vi "TiePie_acq_gen.vi"() -> ()   [LabVIEW 2021]
uses:
  hs3.dll
panel:
  out "Transmitted  Waveform":u16[](graph)
  out "Recieved Samples":i32
  out "Array":string[](array[string])
  out "Recieved Message":string
  in  "Expected Characters":u16
  out "Actual Message Duration":dbl=0.4
  in  "Tranmission Message":string="A"
  in  "Inputs":T1={"Frequency1"=2000.0, "Bit Duration in ms"=0.05, "Frequency2"=4000.0, "Amplitude Scale"=1.0, "Sampling Rate"=50000} {"Frequency2" format="%#_13g"; "Frequency1" format="%#_13g"}
  out "Total Message Duration":dbl=0.4
  in  "Amplitude":dbl(slide)=0.99 min=0.01 max=12.0 step=0.01 scale=0.01..12.0
  in  "Gen_SignalType":u16(ring)=5 caption="Type Signal" items=["Sinus", "Triangle", "Carré", "DC", "Bruit", "Arbitrary"]
  in  "Offset":dbl(slide)=6.661338147750939e-16 min=-12.0 max=12.0 step=0.1 scale=-6.0..6.0
  in  "Démarrer Générateur":bool
  out "Memo untrig":bool
  out "Untrigged":bool
  out "Timebase [s]":dbl=1e-07
  in  "Level [V]":dbl min=-80.0 max=80.0 step=0.001
  in  "Direction":u16(ring) items=["Rising", "Falling"]
  in  "CH1 : AC/DC":u16(ring)=1 items=["AC", "DC"]
  in  "CH2 : AC/DC":u16(ring)=1 items=["AC", "DC"]
  in  "No. of samples":u32=20000 min=100 max=130000 step=1
  in  "Source":u16(ring)=14 items=["CH1"=0, "CH2"=1, "None"=9, "Gen"=14]
  in  "Hysteresis [V]":sgl=0.039997473 min=-100 max=100 step=0.0001 format="%#.4f"
  in  "Active Channel":u16(ring)=1 items=["CH1"=1, "CH2"=2, "CH1 + CH2"=3]
  in  "CH1 Range":dbl(ring)=2.0 items=["200mV"=0.2, "400mV"=0.4, "800mV"=0.8, "2V"=2.0, "4V"=4.0, "8V"=8.0, "20V"=20.0, "40V"=40.0, "80V"=80.0]
  in  "CH2 Range":dbl(ring)=8.0 items=["200mV"=0.2, "400mV"=0.4, "800mV"=0.8, "2V"=2.0, "4V"=4.0, "8V"=8.0, "20V"=20.0, "40V"=40.0, "80V"=80.0]
  in  "Postsamples":i32 min=0 max=130000 step=1
  out "DataReady":bool
  out "Measuring":bool
  in  "Démarrer Acquisition/\nStart Acquisition":bool
  out "Channel B":dbl[](graph)
  out "Channel A":dbl[](graph)
  out "init A":dbl[](array[numeric])
  out "init B":dbl[](array[numeric])
  out "S/N":u32
  out "TiePie OK":bool
  # "General"
  # "Trigger settings"
  # "Canal 1"
  # "Canal 2"
  # "For Debugging"
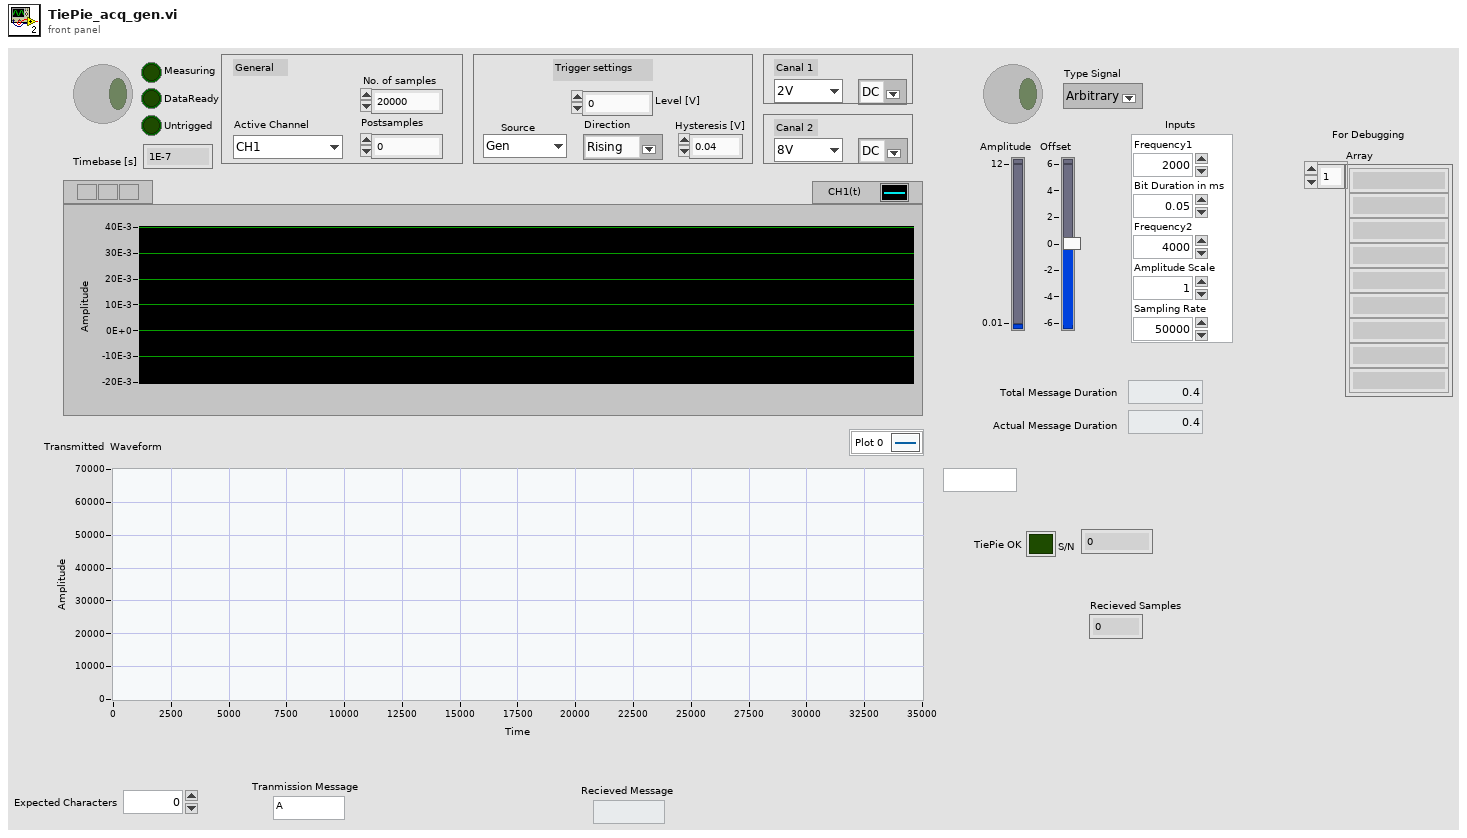
[diagram p1: front panel]
types:
  T1 = cluster{"Frequency1":dbl, "Bit Duration in ms":dbl, "Frequency2":dbl, "Amplitude Scale":dbl, "Sampling Rate":u32}
  T2 = enum8{"Enabled", "Disabled", "Disabled and Grayed Out"}
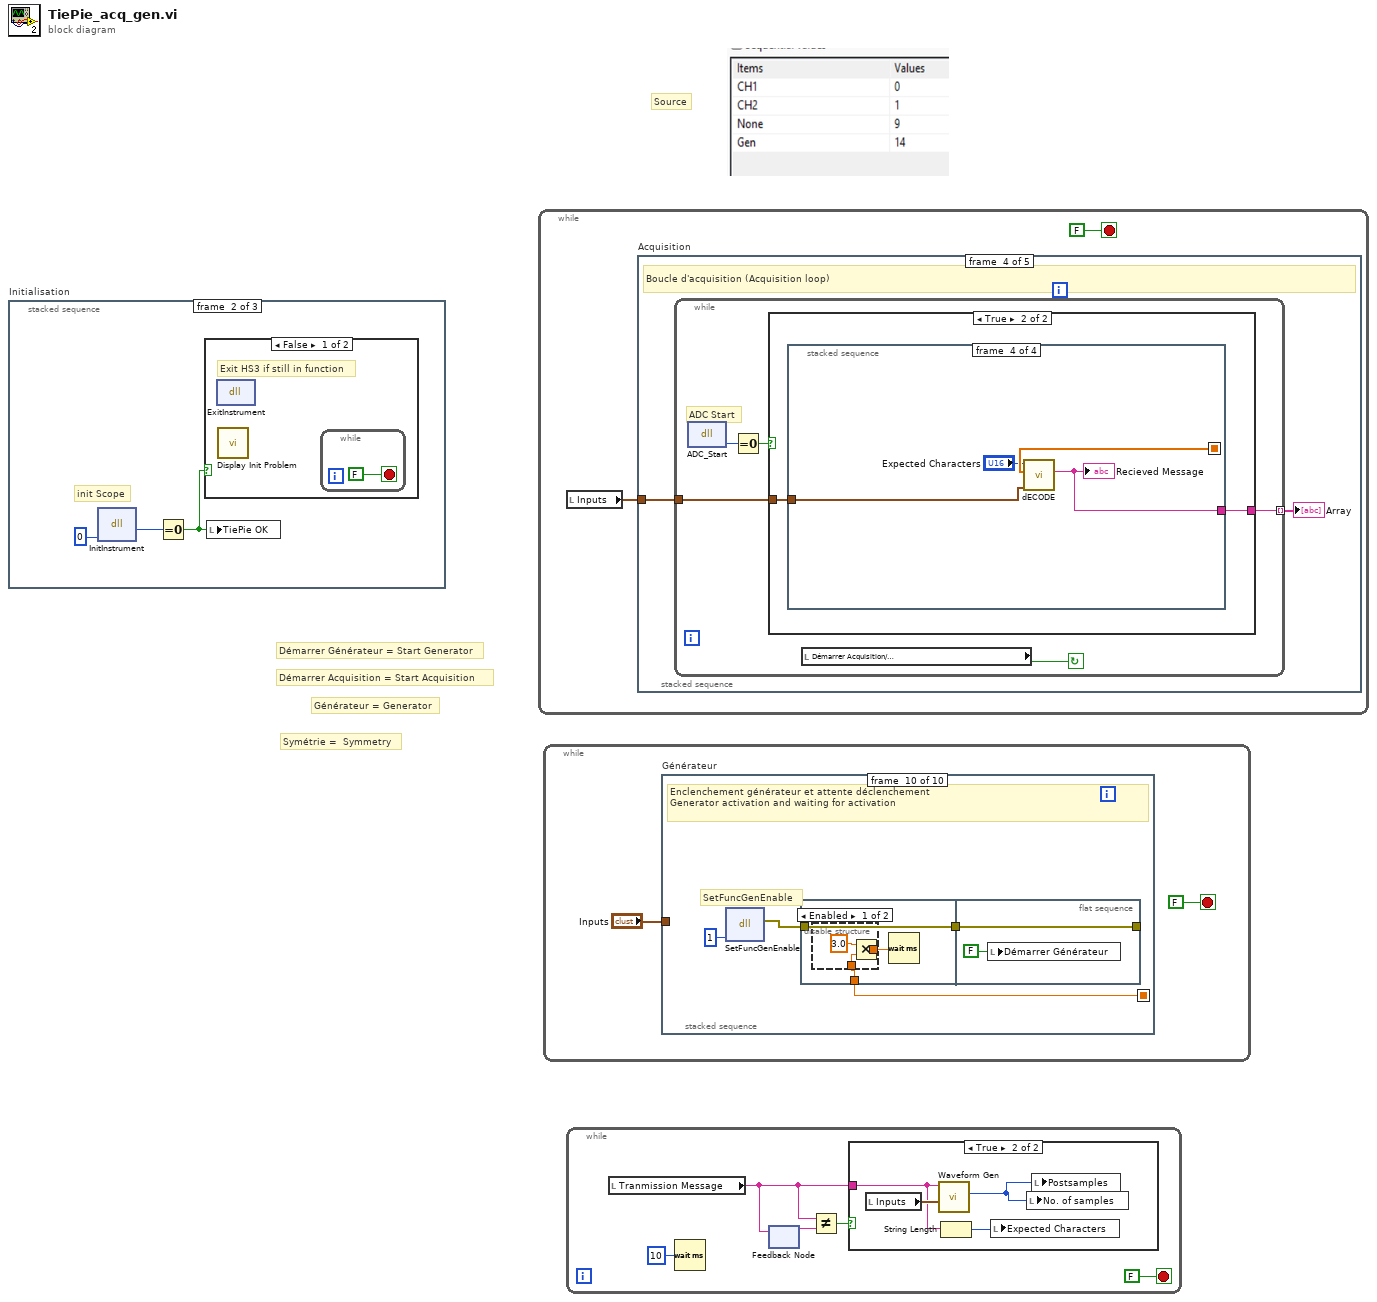
[diagram p0: block diagram]
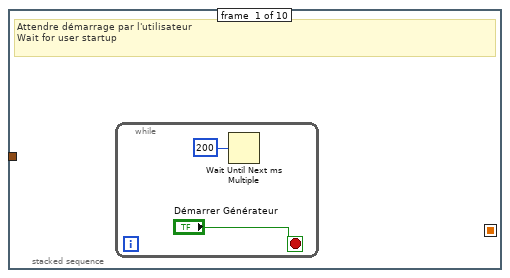
[diagram p3: hidden frame]
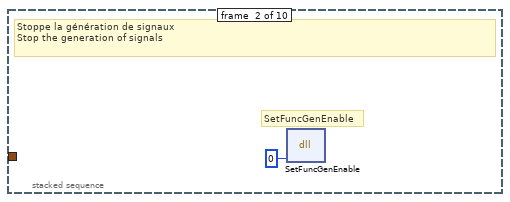
[diagram p4: hidden frame]
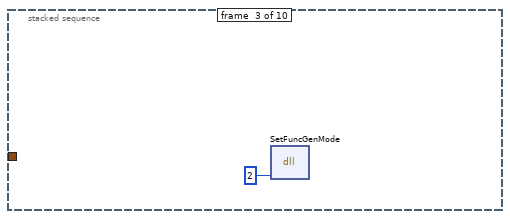
[diagram p5: hidden frame]
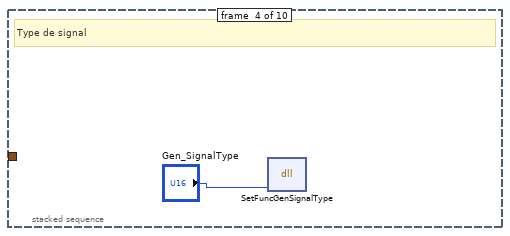
[diagram p6: hidden frame]
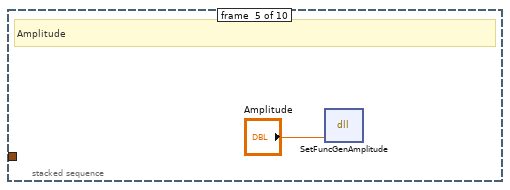
[diagram p7: hidden frame]
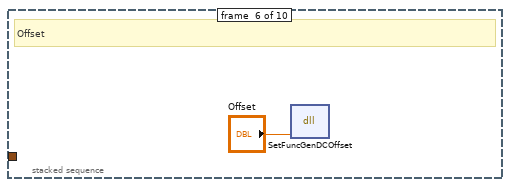
[diagram p8: hidden frame]
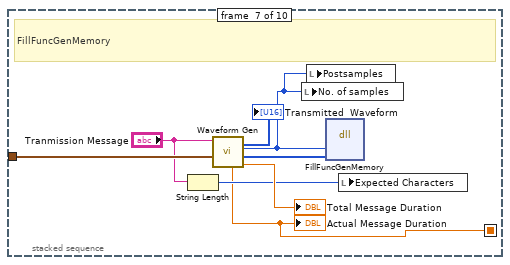
[diagram p9: hidden frame]
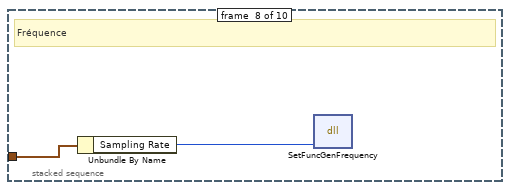
[diagram p10: hidden frame]
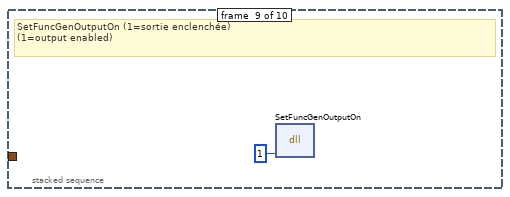
[diagram p11: hidden frame]
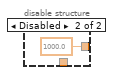
[diagram p12: hidden frame]
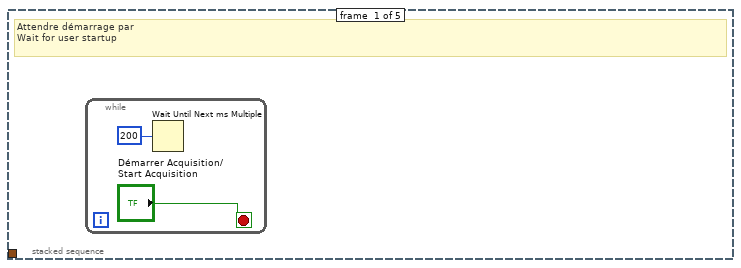
[diagram p13: hidden frame]
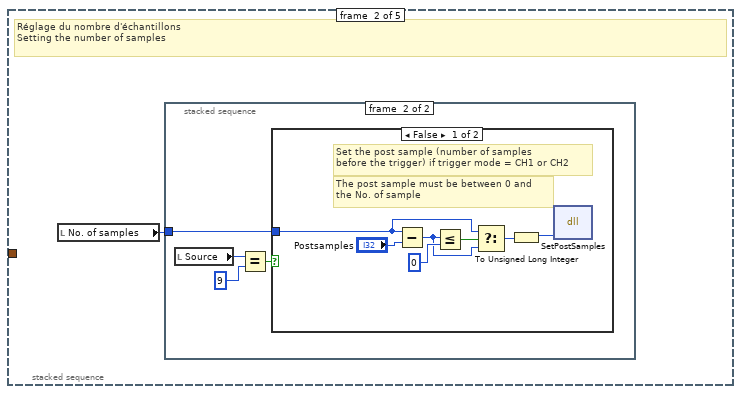
[diagram p14: hidden frame]
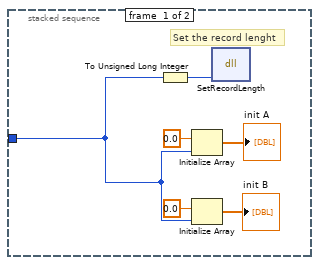
[diagram p15: hidden frame]
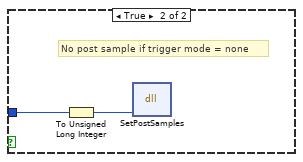
[diagram p16: hidden frame]
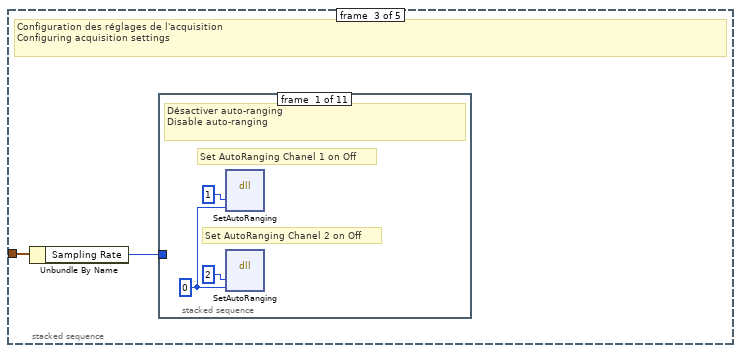
[diagram p17: hidden frame]
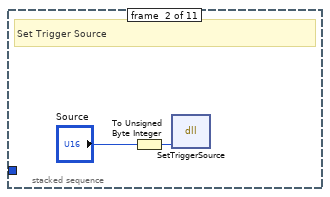
[diagram p18: hidden frame]
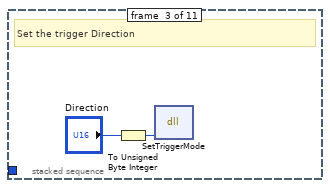
[diagram p19: hidden frame]
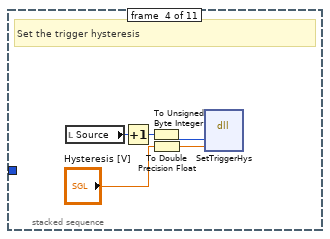
[diagram p20: hidden frame]
diagram:
  # "Source"
  # "Symétrie =  Symmetry"
  # "Générateur = Generator"
  # "Démarrer Acquisition = Start Acquisition"
  # "Démarrer Générateur = Start Generator"
  n1 = stacked-sequence "Initialisation" {
    frame #0 {
      n2 = local write "Démarrer Acquisition/\nStart Acquisition"(FALSE ("Démarrer Acquisition")) -> ()
      n3 = local write "Démarrer Générateur"(FALSE ("Démarrer")) -> ()
      n4 = Wait (ms)(milliseconds to wait=u32 200 ("attente (ms)")) -> ()  [unwired: 1 out]
      n5 = property on="Démarrer Acquisition/\nStart Acquisition" class="Bool (strict)"("DisabledEnum"=T2."Disabled and Grayed Out" ("Désactivé")) -> ()  [unwired: 2 in, 2 out]
      n6 = property on="Démarrer Générateur" class="Bool (strict)"("DisabledEnum"=T2."Disabled and Grayed Out" ("Désactivé")) -> ()  [unwired: 2 in, 2 out]
      "TiePie OK" <- FALSE ("Scope\n init")
      "S/N" <- u32 0 ("Serialnumber")
      "DataReady" <- FALSE ("DataReady")
      "Measuring" <- FALSE ("Measuring")
      "Untrigged" <- FALSE ("Untrigged")
    }
    frame #1 {
      # "init Scope"
      n7 = dll-call lib="C:/Users/BD2QHB4/Desktop/Hassanullah khan/hs3.dll" fn="InitInstrument"("wAddress"=u16 0) -> (w12:u16)  [unwired: 4 in, 2 out]
      n8 = Equal To 0?(x=w12) -> (x = 0?=w11:bool)
      n9 = case shown="False" w11 {
        frame False {
          # "Exit HS3 if still in function"
          n10 = dll-call lib="C:/Users/BD2QHB4/Desktop/Hassanullah khan/hs3.dll" fn="ExitInstrument"() -> ()  [unwired: 4 in, 2 out]
          n11 = call "Display Init Problem"() -> ()  [unwired: 10 in, 2 out]
          n12 = while {
            stop <- FALSE stop-if-true
          }
        }
        frame True {
        }
      }
      n13 = local write "TiePie OK"(w11) -> ()
    }
    frame #2 {
      n14 = local read "S/N"() -> (w17:u32)
      n15 = property on="Démarrer Acquisition/\nStart Acquisition" class="Bool (strict)"("DisabledEnum"=T2."Enabled" ("Désactivé")) -> ()  [unwired: 2 in, 2 out]
      n16 = property on="Démarrer Générateur" class="Bool (strict)"("DisabledEnum"=T2."Enabled" ("Désactivé")) -> ()  [unwired: 2 in, 2 out]
      n17 = dll-call lib="C:/Users/BD2QHB4/Desktop/Hassanullah khan/hs3.dll" fn="GetSerialNumber"("dwSerialNumber"=w17) -> ("dwSerialNumber"=w18:u32)  [unwired: 4 in, 2 out]
      n18 = local write "S/N"(w18) -> ()
    }
  }
  n19 = while {
    stop <- FALSE stop-if-true
    n20 = local read "Inputs"() -> (w19:T1)
    n21 = stacked-sequence "Acquisition" {
      tunnel: w19 -> [_ _ w44 w81 _]
      frame #0 {
        # "Attendre démarrage par \nWait for user startup"
        n22 = while {
          stop <- "Démarrer Acquisition/\nStart Acquisition" stop-if-true
          n23 = Wait Until Next ms Multiple(millisecond multiple=u32 200) -> ()  [unwired: 1 out]
        }
      }
      frame #1 {
        # "Réglage du nombre d'échantillons\nSetting the number of samples"
        n24 = local read "No. of samples"() -> (w23:u32)
        n25 = stacked-sequence {
          tunnel: w23 -> [w24 w30]
          frame #0 {
            # "Set the record lenght"
            n26 = To Unsigned Long Integer(number=w24) -> (unsigned 32bit integer=w29:u32)
            n27 = Initialize Array(0.0, w24) -> (→"init A":dbl[])
            n28 = Initialize Array(0.0, w24) -> (→"init B":dbl[])
            n29 = dll-call lib="C:/Users/BD2QHB4/Desktop/Hassanullah khan/hs3.dll" fn="SetRecordLength"("dTotal"=w29) -> ()  [unwired: 5 in, 2 out]
          }
          frame #1 {
            n30 = local read "Source"() -> (w33:u16)
            n31 = Equal?(x=w33, y=u16 9) -> (x = y?=w31:bool)
            n32 = case shown="False" w31 {
              tunnel: w30 -> [w36 w42]
              frame False {
                # "The post sample must be between 0 and \nthe No. of sample"
                # "Set the post sample (number of samples\nbefore the trigger) if trigger mode = CH1 or CH2"
                n33 = Subtract(x=w36, y="Postsamples") -> (x-y=w35:u32)
                n34 = Less Or Equal?(x=w35, y=0) -> (x <= y?=w37:bool)
                n35 = Select(t=w36, s=w37, f=w35) -> (s? t:f=w39:u32)
                n36 = To Unsigned Long Integer(number=w39) -> (unsigned 32bit integer=w40:u32)
                n37 = dll-call lib="C:/Users/BD2QHB4/Desktop/Hassanullah khan/hs3.dll" fn="SetPostSamples"("dTotal"=w40) -> ()  [unwired: 5 in, 2 out]
              }
              frame True {
                # "No post sample if trigger mode = none"
                n38 = To Unsigned Long Integer(number=w42) -> (unsigned 32bit integer=w41:u32)
                n39 = dll-call lib="C:/Users/BD2QHB4/Desktop/Hassanullah khan/hs3.dll" fn="SetPostSamples"("dTotal"=w41) -> ()  [unwired: 5 in, 2 out]
              }
            }
          }
        }
      }
      frame #2 {
        # "Configuration des réglages de l'acquisition\nConfiguring acquisition settings"
        n40 = Unbundle By Name(w44) -> ("Sampling Rate"=w43:u32)
        n41 = stacked-sequence {
          tunnel: w43 -> [_ _ _ _ _ _ _ _ _ _ w76]
          frame #0 {
            w47 = u8 0
            # "Set AutoRanging Chanel 1 on Off"
            # "Set AutoRanging Chanel 2 on Off"
            # "Désactiver auto-ranging\nDisable auto-ranging"
            n42 = dll-call lib="C:/Users/BD2QHB4/Desktop/Hassanullah khan/hs3.dll" fn="SetAutoRanging"("byCh"=u8 1, "byMode"=w47) -> ()  [unwired: 6 in, 2 out]
            n43 = dll-call lib="C:/Users/BD2QHB4/Desktop/Hassanullah khan/hs3.dll" fn="SetAutoRanging"("byCh"=u8 2, "byMode"=w47) -> ()  [unwired: 6 in, 2 out]
          }
          frame #1 {
            # "Set Trigger Source"
            n44 = To Unsigned Byte Integer(number="Source") -> (unsigned 8bit integer=w49:u8)
            n45 = dll-call lib="C:/Users/BD2QHB4/Desktop/Hassanullah khan/hs3.dll" fn="SetTriggerSource"("byTrigSource"=w49) -> ()  [unwired: 5 in, 2 out]
          }
          frame #2 {
            # "Set the trigger Direction"
            n46 = To Unsigned Byte Integer(number="Direction") -> (unsigned 8bit integer=w51:u8)
            n47 = dll-call lib="C:/Users/BD2QHB4/Desktop/Hassanullah khan/hs3.dll" fn="SetTriggerMode"("byTrigMode"=w51) -> ()  [unwired: 5 in, 2 out]
          }
          frame #3 {
            # "Set the trigger hysteresis"
            n48 = local read "Source"() -> (w55:u16)
            n49 = Increment(x=w55) -> (x+1=w53:u16)
            n50 = To Unsigned Byte Integer(number=w53) -> (unsigned 8bit integer=w56:u8)
            n51 = To Double Precision Float(number="Hysteresis [V]") -> (double precision float=w54:dbl)
            n52 = dll-call lib="C:/Users/BD2QHB4/Desktop/Hassanullah khan/hs3.dll" fn="SetTriggerHys"("byCh"=w56, "rHysteresis"=w54) -> ()  [unwired: 6 in, 2 out]
          }
          frame #4 {
            # "Set the trigger Level"
            n53 = local read "Source"() -> (w60:u16)
            n54 = Increment(x=w60) -> (x+1=w58:u16)
            n55 = To Unsigned Byte Integer(number=w58) -> (unsigned 8bit integer=w61:u8)
            n56 = To Double Precision Float(number="Level [V]") -> (double precision float=w59:dbl)
            n57 = dll-call lib="C:/Users/BD2QHB4/Desktop/Hassanullah khan/hs3.dll" fn="SetTriggerLevel"("byCh"=w61, "rLvl"=w59) -> ()  [unwired: 6 in, 2 out]
          }
          frame #5 {
            # "Set the mesure mode (Source)"
            n58 = To Unsigned Byte Integer(number="Active Channel") -> (unsigned 8bit integer=w63:u8)
            n59 = dll-call lib="C:/Users/BD2QHB4/Desktop/Hassanullah khan/hs3.dll" fn="SetMeasureMode"("byMode"=w63) -> ()  [unwired: 5 in, 2 out]
          }
          frame #6 {
            # "Set the channel 1 Range"
            n60 = To Double Precision Float(number="CH1 Range") -> (double precision float=w66:dbl)
            n61 = dll-call lib="C:/Users/BD2QHB4/Desktop/Hassanullah khan/hs3.dll" fn="SetSensitivity"("byCh"=u8 1, "rSens"=w66) -> ()  [unwired: 6 in, 2 out]
          }
          frame #7 {
            # "Set the channel 2 Range"
            n62 = To Double Precision Float(number="CH2 Range") -> (double precision float=w68:dbl)
            n63 = dll-call lib="C:/Users/BD2QHB4/Desktop/Hassanullah khan/hs3.dll" fn="SetSensitivity"("byCh"=u8 2, "rSens"=w68) -> ()  [unwired: 6 in, 2 out]
          }
          frame #8 {
            # "Set the coupling CH1"
            n64 = To Unsigned Byte Integer(number="CH1 : AC/DC") -> (unsigned 8bit integer=w71:u8)
            n65 = dll-call lib="C:/Users/BD2QHB4/Desktop/Hassanullah khan/hs3.dll" fn="SetCoupling"("byCh"=u8 1, "byMode"=w71) -> ()  [unwired: 6 in, 2 out]
          }
          frame #9 {
            # "Set the coupling CH2"
            n66 = To Unsigned Byte Integer(number="CH2 : AC/DC") -> (unsigned 8bit integer=w75:u8)
            n67 = dll-call lib="C:/Users/BD2QHB4/Desktop/Hassanullah khan/hs3.dll" fn="SetCoupling"("byCh"=u8 2, "byMode"=w75) -> ()  [unwired: 6 in, 2 out]
          }
          frame #10 {
            # "Set the sample frequency"
            n68 = To Unsigned Long Integer(number=w76) -> (unsigned 32bit integer=w79:u32)
            n69 = dll-call lib="C:/Users/BD2QHB4/Desktop/Hassanullah khan/hs3.dll" fn="SetSampleFrequency"("dFreq"=w79) -> ("dFreq"=w78:u32)  [unwired: 4 in, 2 out]
            n70 = Reciprocal(x=w78) -> (1/x=w77:dbl)
            "Timebase [s]" <- w77
            n71 = property on="Channel A" class="WFGraph (strict)"("XScale.Multiplier"=w77) -> ()  [unwired: 2 in, 2 out]
            n72 = property on="Channel B" class="WFGraph (strict)"("XScale.Multiplier"=w77) -> ()  [unwired: 2 in, 2 out]
          }
        }
      }
      frame #3 {
        # "Boucle d'acquisition (Acquisition loop)"
        n73 = while {
          tunnel: w81 -> [w83]
          tunnel: [w82] -> w80 mode=indexing
          stop <- w84 continue-if-true
          # "ADC Start"
          n74 = dll-call lib="C:/Users/BD2QHB4/Desktop/Hassanullah khan/hs3.dll" fn="ADC_Start"() -> (w86:u16)  [unwired: 3 in, 2 out]
          n75 = Equal To 0?(x=w86) -> (x = 0?=w85:bool)
          n76 = case shown="True" w85 {
            tunnel: w83 -> [_ w89]
            tunnel: [_ w88] -> w82
            frame False {
              # "ACQ problem display"
              n77 = call "Affiche problème ACQ"() -> ()  [unwired: 10 in, 2 out]
              n78 = while {
                stop <- FALSE stop-if-true
              }
            }
            frame True {
              n79 = stacked-sequence {
                seq-local: [_ _ w104 _] -> [_ _ _ w112]
                tunnel: w89 -> [_ _ _ w110]
                tunnel: [_ _ _ w109] -> w88
                frame #0 {
                  # "ADC_Running"
                  # "Mesure en cours\nAction in progress"
                  n80 = dll-call lib="C:/Users/BD2QHB4/Desktop/Hassanullah khan/hs3.dll" fn="ADC_Running"() -> ("type de retour"=w93:u16)  [unwired: 3 in, 2 out]
                  n81 = Equal?(x=u16 1, y=w93) -> (x = y?=w92:bool)
                  n82 = local write "Measuring"(w92) -> ()
                  "Memo untrig" <- FALSE ("Memo untrig")
                }
                frame #1 {
                  # "Attendre mesure prête (ou timeout trigger)\nWait for measurement ready (or timeout trigger)"
                  n83 = while {
                    i -> [w98]
                    stop <- w95 stop-if-true
                    n84 = Equal To 0?(x=w98) -> (x = 0?=w97:bool)
                    n85 = call "Temps écoulé"("Time Target (s)"=1.0, "Reset"=w97, "Auto Reset"=FALSE) -> ("Time has Elapsed"=w94:bool)  [unwired: 9 in, 7 out]
                    n86 = case shown="True" w94 {
                      selector: w94 -> [w102 _]
                      frame True {
                        # "Force Trig"
                        n87 = dll-call lib="C:/Users/BD2QHB4/Desktop/Hassanullah khan/hs3.dll" fn="ADC_ForceTrig"() -> ()  [unwired: 4 in, 2 out]
                        n88 = local write "Memo untrig"(w102) -> ()
                      }
                      frame False {
                      }
                    }
                    n89 = dll-call lib="C:/Users/BD2QHB4/Desktop/Hassanullah khan/hs3.dll" fn="ADC_Ready"() -> (w96:u16)  [unwired: 3 in, 2 out]
                    n90 = Greater Than 0?(x=w96) -> (x > 0?=w95:bool)
                    n91 = local write "DataReady"(w95) -> ()
                    n92 = Wait Until Next ms Multiple(millisecond multiple=u32 5) -> ()  [unwired: 1 out]
                  }
                }
                frame #2 {
                  # "Get ADC Value in Volt"
                  # "Récupération des valeurs\nRetrieving values"
                  n93 = local read "Memo untrig"() -> (w105:bool)
                  n94 = local read "init A"() -> (w107:dbl[])
                  n95 = local read "init B"() -> (w108:dbl[])
                  n96 = local write "Untrigged"(w105) -> ()
                  n97 = dll-call lib="C:/Users/BD2QHB4/Desktop/Hassanullah khan/hs3.dll" fn="ADC_GetDataVolt"("dCh1"=w107, "dCh2"=w108) -> ("dCh1"=w104:dbl[], "dCh2"=→"Channel B":dbl[])  [unwired: 4 in, 2 out]
                  "Channel A" <- w104
                  n98 = Array Size(array=w104) -> (size(s)=→"Recieved Samples":i32)
                }
                frame #3 {
                  n99 = call "dECODE.vi"("Inputs"=w110, "Waveform Array"=w112, "Expected Characters"="Expected Characters") -> ("string"=w109:string)  [unwired: 8 in]
                  "Recieved Message" <- w109
                }
              }
            }
          }
          n100 = local read "Démarrer Acquisition/\nStart Acquisition"() -> (w84:bool)
        }
        "Array" <- w80
      }
      frame #4 {
        # "ADC_Running"
        # "ADC_abort"
        # "Stoppe l'acquisition\nStop the acquisition"
        n101 = dll-call lib="C:/Users/BD2QHB4/Desktop/Hassanullah khan/hs3.dll" fn="ADC_Running"() -> ("type de retour"=w114:u16)  [unwired: 3 in, 2 out]
        n102 = dll-call lib="C:/Users/BD2QHB4/Desktop/Hassanullah khan/hs3.dll" fn="ADC_Abort"() -> ()  [unwired: 4 in, 2 out]
        n103 = Equal?(x=u16 1, y=w114) -> (x = y?=w115:bool)
        n104 = local write "DataReady"(FALSE ("DataReady")) -> ()
        n105 = local write "Measuring"(w115) -> ()
      }
    }
  }
  n106 = while {
    stop <- FALSE stop-if-true
    n107 = stacked-sequence "Générateur" {
      seq-local: [_ _ _ _ _ _ w126 _ _ _] -> [_ _ _ _ _ _ _ _ _ w137]
      tunnel: "Inputs" -> [_ _ _ _ _ _ w132 w135 _ _]
      frame #0 {
        # "Attendre démarrage par l'utilisateur\nWait for user startup"
        n108 = while {
          stop <- "Démarrer Générateur" stop-if-true
          n109 = Wait Until Next ms Multiple(millisecond multiple=u32 200) -> ()  [unwired: 1 out]
        }
      }
      frame #1 {
        # "SetFuncGenEnable"
        # "Stoppe la génération de signaux\nStop the generation of signals"
        n110 = dll-call lib="C:/Users/BD2QHB4/Desktop/Hassanullah khan/hs3.dll" fn="SetFuncGenEnable"("arg1"=u16 0) -> ()  [unwired: 5 in, 2 out]
      }
      frame #2 {
        n111 = dll-call lib="C:/Users/BD2QHB4/Desktop/Hassanullah khan/hs3.dll" fn="SetFuncGenMode"("dwMode"=2) -> ()  [unwired: 5 in, 2 out]
      }
      frame #3 {
        # "Type de signal"
        n112 = dll-call lib="C:/Users/BD2QHB4/Desktop/Hassanullah khan/HS3.dll" fn="SetFuncGenSignalType"("SignalType"="Gen_SignalType") -> ()  [unwired: 5 in, 2 out]
      }
      frame #4 {
        # "Amplitude"
        n113 = dll-call lib="C:/Users/BD2QHB4/Desktop/Hassanullah khan/hs3.dll" fn="SetFuncGenAmplitude"("Amplitude") -> ()  [unwired: 5 in, 2 out]
      }
      frame #5 {
        # "Offset"
        n114 = dll-call lib="C:/Users/BD2QHB4/Desktop/Hassanullah khan/HS3.dll" fn="SetFuncGenDCOffset"("Offset") -> ()  [unwired: 5 in, 2 out]
      }
      frame #6 {
        # "FillFuncGenMemory"
        n115 = String Length(string="Tranmission Message") -> (length=w128:i32)
        n116 = call "Waveform Gen.vi"("Inputs"=w132, "Message String"="Tranmission Message") -> ("Total Message Duration"=→"Total Message Duration":dbl, "Waveform Array"=w131:u16[], "No. of Points"=w130:u64, "Actual Message Duration"=w126:dbl, "Waveform Graph"=→"Transmitted  Waveform":u16[])  [unwired: 5 in]
        "Actual Message Duration" <- w126
        n117 = local write "No. of samples"(w130) -> ()
        n118 = local write "Postsamples"(w130) -> ()
        n119 = dll-call lib="C:/Users/BD2QHB4/Desktop/Hassanullah khan/hs3.dll" fn="FillFuncGenMemory" label="SetFuncGenMode"("dwNrPoints"=w130, "wFuncGenData"=w131) -> ()  [unwired: 6 in, 2 out]
        n120 = local write "Expected Characters"(w128) -> ()
      }
      frame #7 {
        # "Fréquence"
        n121 = Unbundle By Name(w135) -> ("Sampling Rate"=w134:u32)
        n122 = dll-call lib="C:/Users/BD2QHB4/Desktop/Hassanullah khan/hs3.dll" fn="SetFuncGenFrequency"(w134) -> ()  [unwired: 5 in, 2 out]
      }
      frame #8 {
        # "SetFuncGenOutputOn (1=sortie enclenchée)\n(1=output enabled)"
        n123 = dll-call lib="C:/Users/BD2QHB4/Desktop/Hassanullah khan/hs3.dll" fn="SetFuncGenOutputOn"("arg1"=u16 1) -> ()  [unwired: 5 in, 2 out]
      }
      frame #9 {
        # "SetFuncGenEnable"
        # "Enclenchement générateur et attente déclenchement\nGenerator activation and waiting for activation"
        n124 = dll-call lib="C:/Users/BD2QHB4/Desktop/Hassanullah khan/hs3.dll" fn="SetFuncGenEnable"("arg1"=u16 1) -> (error out=w139:errorcluster)  [unwired: 5 in, 1 out]
        n125 = flat-sequence {
          tunnel: w139 -> [w143]
          tunnel: [w143] -> w138
          tunnel: w137 -> [w142]
          tunnel: [w149] -> _
          tunnel: w138 -> [w149]
          frame #0 {
            n126 = disable-structure shown="Enabled" {
              disable-tunnel: w142 -> [w146 _]
              disable-tunnel: [w144 1000.0] -> w141
              frame Enabled {
                n127 = Multiply(x=3.0, y=w146) -> (x*y=w144:dbl)
              }
              frame Disabled {
              }
            }
            n128 = Wait (ms)(milliseconds to wait=w141) -> ()  [unwired: 1 out]
          }
          frame #1 {
            n129 = local write "Démarrer Générateur"(FALSE ("Démarrer Générateur")) -> ()
          }
        }
      }
    }
  }
  n130 = while {
    stop <- FALSE stop-if-true
    n131 = local read "Tranmission Message"() -> (w150:string)
    n132 = Wait (ms)(milliseconds to wait=u32 10) -> ()  [unwired: 1 out]
    n133 = feedback-in #1(w150) -> ()
    n134 = feedback #1() -> (w154:string)  [unwired: 1 in]
    n135 = Not Equal?(x=w150, y=w154) -> (x != y?=w153:bool)
    n136 = case shown="True" w153 {
      tunnel: w150 -> [_ w156]
      frame False {
      }
      frame True {
        n137 = local read "Inputs"() -> (w158:T1)
        n138 = call "Waveform Gen.vi"("Inputs"=w158, "Message String"=w156) -> ("No. of Points"=w157:u64)  [unwired: 5 in, 4 out]
        n139 = String Length(string=w156) -> (length=w155:i32)
        n140 = local write "Expected Characters"(w155) -> ()
        n141 = local write "No. of samples"(w157) -> ()
        n142 = local write "Postsamples"(w157) -> ()
      }
    }
  }
